vi "Unit Test Allow Non-BlueSerializable Objects True.vi"() -> ()   [LabVIEW 2019, in "Sports Unit Tests.lvclass"]
uses:
  Sports Unit Tests.lvclass
  Classes/NonBlueSerializable/NonBlueSerializable.lvclass
  <userlib>/Blue Origin/BlueSerialization/BlueSerializer/SerializeOptions.ctl
  <userlib>/Blue Origin/BlueSerialization/BlueSerializer/DeserializeOptions.ctl
  <userlib>/Blue Origin/BlueSerialization/BlueSerializer/DeserializeSlicingOptions.ctl
  <userlib>/Blue Origin/BlueSerialization/BlueSerializer/DeserializeMutationOptions.ctl
  <userlib>/Blue Origin/BlueSerialization/BlueSerializer/DeserializePreservationOptions.ctl
  <userlib>/Blue Origin/BlueSerialization/BlueSerializer/PreserveNonWiredDataOption.ctl
  Classes/NonBlueSerializable/NonBlueSerializable.lvclass/NonBlueSerializable.ctl
  Classes/NonBlueSerializable/Write Boolean.vi
  Classes/NonBlueSerializable/Write Numeric.vi
  Classes/NonBlueSerializable/Write String.vi
  <vilib>/Utility/error.llb/Clear Errors.vi
  <vilib>/addons/_JKI Toolkits/Caraya/classes/Test/Define Test.vi
  <vilib>/addons/_JKI Toolkits/Caraya/classes/Assert/Assert Equal Value_Variant.vi
  <vilib>/addons/_JKI Toolkits/Caraya/classes/Assert/Assert Not Error.vi
  <vilib>/addons/_JKI Toolkits/Caraya/classes/Assert/Assert.lvclass
  <userlib>/Blue Origin/BlueSerialization/BlueSerializer/BlueSerializer.lvclass
panel:
  out "Table":string[][](table)
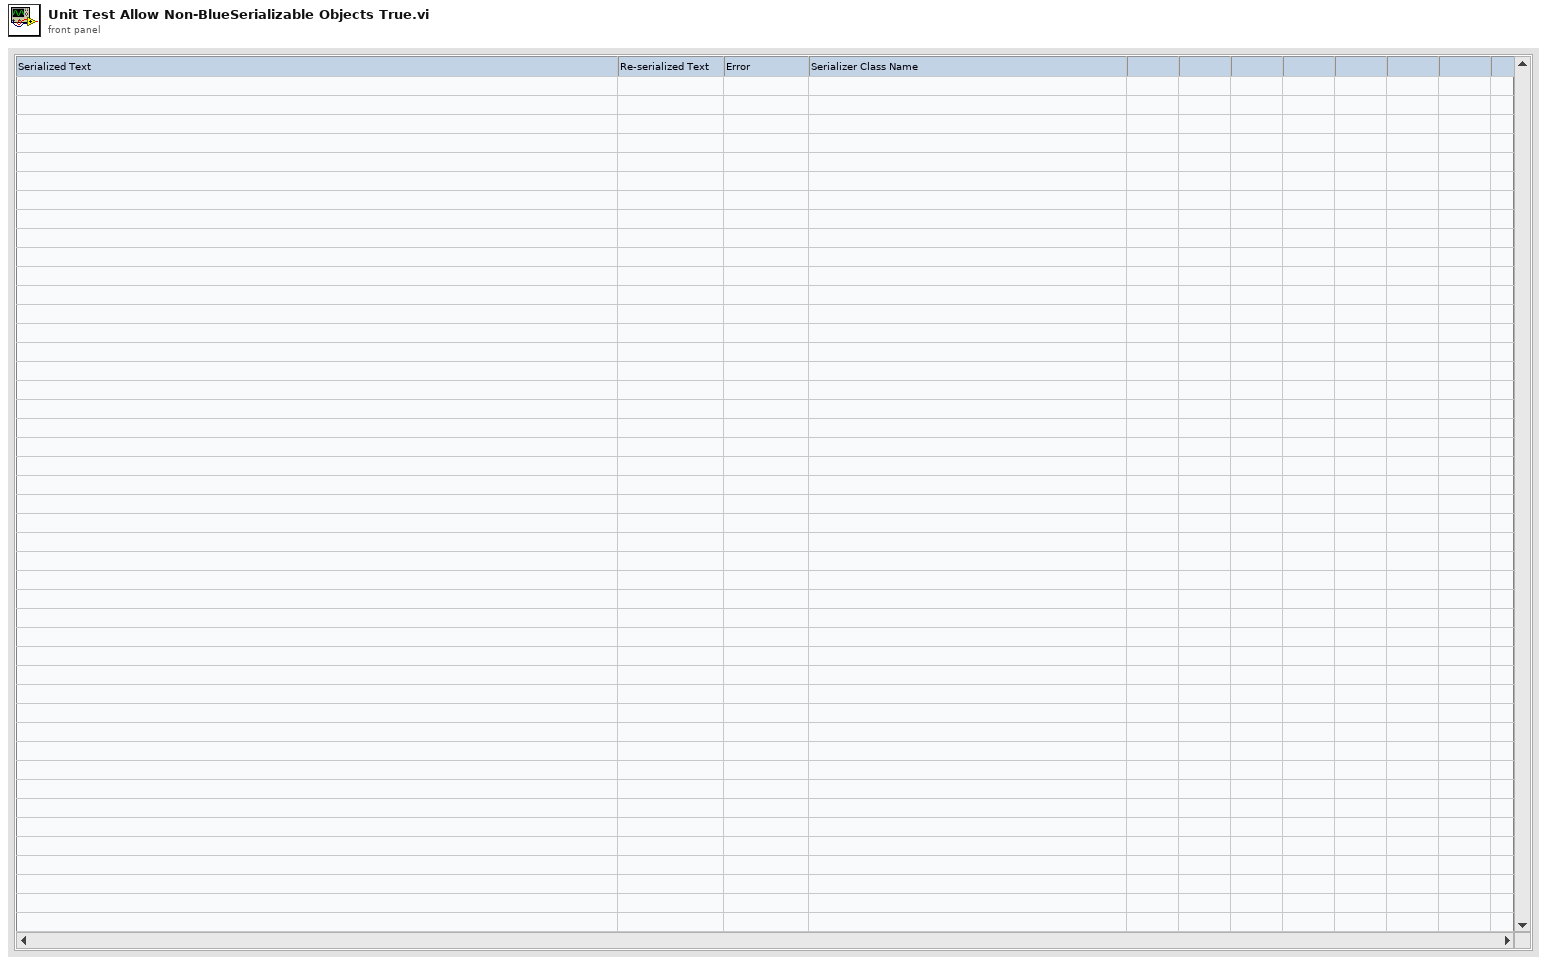
[diagram p1: front panel]
types:
  T1 = typedef "BlueSerialization.lvlib/BlueSerializer.lvclass/DeserializeOptions.ctl" = cluster{"deserialize non-BlueSerializable objects from hex?":bool, "expand objects on type conflict?":bool, "Slicing":T2, "Mutation Options":T3, "Preservation Options":T4}
  T2 = typedef "BlueSerialization.lvlib/BlueSerializer.lvclass/DeserializeSlicingOptions.ctl" = cluster{"slice flattened object data on error?":bool, "sliceable class names":string[]}
  T3 = typedef "BlueSerialization.lvlib/BlueSerializer.lvclass/DeserializeMutationOptions.ctl" = cluster{"error on inserted parent levels?":bool, "\terror on obsolete parent levels?":bool}
  T4 = typedef "BlueSerialization.lvlib/BlueSerializer.lvclass/DeserializePreservationOptions.ctl" = cluster{"Preserve wired serialized data?":bool, "Preserve wired non-serialized data":T5}
  T5 = typedef "BlueSerialization.lvlib/BlueSerializer.lvclass/PreserveNonWiredDataOption.ctl" = enum16{"Don't preserve", "Preserve (error on less-specific wired types)", "Preserve (except on less-specific wired types)"}
  T6 = typedef "BlueSerialization.lvlib/BlueSerializer.lvclass/SerializeOptions.ctl" = cluster{"serialize non-BlueSerializable objects as hex?":bool, "slice objects per SetSerializeSliceClass.vi?":bool}
  T7 = cluster{"NonBlueSerializable.lvclass":refnum<class "NonBlueSerializable.lvclass">}
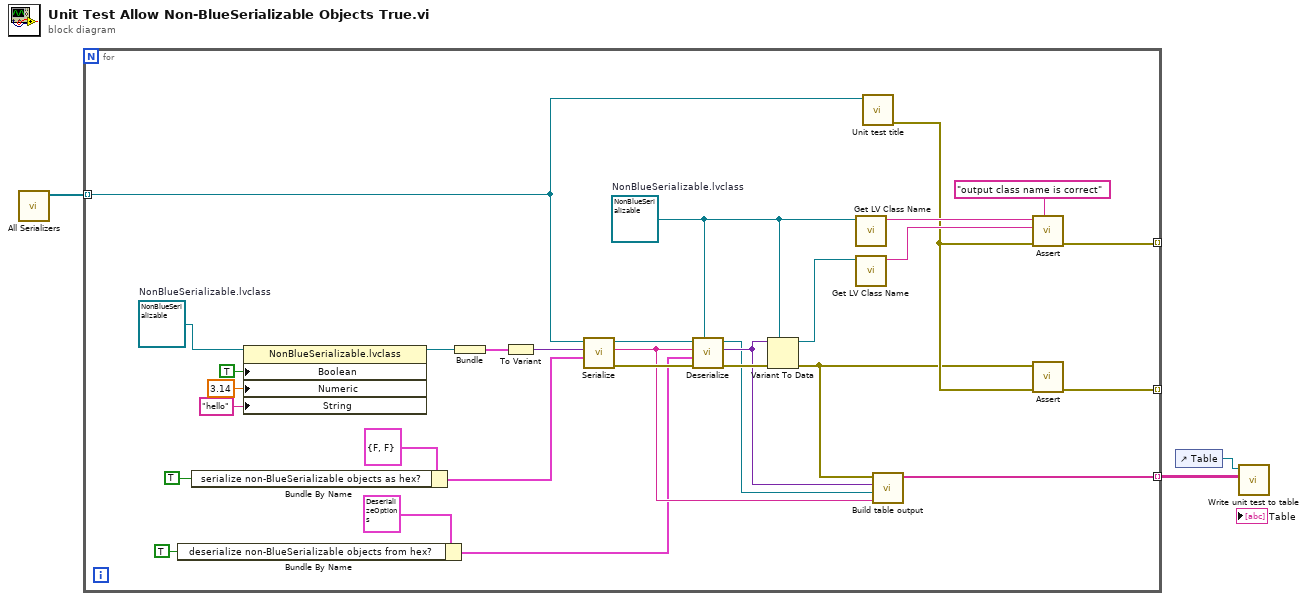
[diagram p0: block diagram]
diagram:
  n1 = call "All Serializers.vi"() -> ("All serializers"=w1:refnum<class "BlueSerializer.lvclass">[])  [unwired: 11 in]
  n2 = for {
    tunnel: w1 -> [w6] mode=indexing
    tunnel: [w17] -> w3 mode=indexing
    tunnel: [w25] -> _ mode=indexing
    tunnel: [w24] -> _ mode=indexing
    w18 = refnum<class "NonBlueSerializable.lvclass"> refnum  # NonBlueSerializable.lvclass
    w22 = refnum<class "NonBlueSerializable.lvclass"> refnum  # NonBlueSerializable.lvclass
    n3 = Bundle By Name(cluster=T1 {"deserialize non-BlueSerializable objects from hex?"=FALSE, "expand objects on type conflict?"=FALSE, "Slicing"={"slice flattened object data on error?"=FALSE, "sliceable class names"=[]}, "Mutation Options"={"error on inserted parent levels?"=FALSE, "\terror on obsolete parent levels?"=FALSE}, "Preservation Options"={"Preserve wired serialized data?"=FALSE, "Preserve wired non-serialized data"=enum."Don't preserve"}} ("Deserialize Options"), "deserialize non-BlueSerializable objects from hex?"=TRUE ("Allow non-BlueSerializable objects?")) -> (w4:T1)
    n4 = Bundle By Name(cluster=T6 {"serialize non-BlueSerializable objects as hex?"=FALSE, "slice objects per SetSerializeSliceClass.vi?"=FALSE} ("Serialize Options"), "serialize non-BlueSerializable objects as hex?"=TRUE ("Allow class slicing?")) -> (w5:T6)
    n5 = property on="Property Node" class="NonBlueSerializable.lvclass"(reference=w22, "Boolean"=TRUE, "Numeric"=3.14, "String"="hello") -> (reference out=w12:refnum<class "NonBlueSerializable.lvclass">)  [unwired: 1 in, 1 out]
    n6 = Bundle("NonBlueSerializable.lvclass"=w12) -> (w11:T7)  [unwired: 1 in]
    n7 = To Variant(anything=w11) -> (Variant=w31:variant)
    n8 = call <userlib>:"Serialize.vi"("Serialize Options"=w5, "Anything"=w31, "BlueSerializer in"=w6) -> ("error out"=w33:errorcluster, "Serialized Text"=w13:string, "BlueSerializer out"=w32:refnum<class "BlueSerializer.lvclass">)  [unwired: 6 in]
    n9 = call <userlib>:"Deserialize.vi"("Anything"=w18, "error in (no error)"=w33, "Deserialize Options"=w4, "Serialized Text"=w13, "BlueSerializer in"=w32) -> ("error out"=w30:errorcluster, "Variant"=w15:variant, "BlueSerializer out"=w14:refnum<class "BlueSerializer.lvclass">)  [unwired: 4 in]
    n10 = Variant To Data(error in=w30, type=w18, Variant=w15) -> (data=w29:refnum<class "NonBlueSerializable.lvclass">, error out=w16:errorcluster)
    n11 = call <vilib>:"Get LV Class Name.vi"("object"=w18) -> ("class name"=w28:string)  [unwired: 9 in, 1 out]
    n12 = call <vilib>:"Get LV Class Name.vi"("object"=w29) -> ("class name"=w27:string)  [unwired: 9 in, 1 out]
    n13 = call "Unit test title.vi"("serializer"=w6) -> ("error out"=w23:errorcluster)  [unwired: 9 in, 1 out]
    n14 = call "Build table output.vi"("serialized text"=w13, "BlueSerializer in"=w14, "deserialized variant"=w15, "variant to data error"=w16) -> ("table output"=w17:string[])  [unwired: 7 in]
    n15 = call-poly <vilib>:"Assert.vi"("Label"="output class name is correct", "error in (no error)"=w23, "Y"=w27, "X"=w28) -> ("error out"=w24:errorcluster)  [unwired: 7 in]
    n16 = call-poly <vilib>:"Assert.vi"("error in (no error)"=w23, "Not Error?"=w16) -> ("error out"=w25:errorcluster)  [unwired: 9 in]
  }
  n17 = control-ref of="Table"() -> (w2:refnum<vi>)
  n18 = call "Write unit test to table.vi"("Table"=w3, "Table ref in"=w2) -> ()  [unwired: 9 in, 1 out]
